vi "Memory Management.MoveDblBlock.Write (Double).vi"(0 "src ptr in":u64, 1 "src offset (0)":u64, 2 "dst in":dbl[](array[numeric]), 3 "dst index (0)":u64, 4 "count":u64, 5 "error in (no error)":errorcluster) -> (14 "src ptr out":u64, 15 "src offset out":u64, 16 "dst out":dbl[](array[numeric]), 17 "dst index out":u64, 18 "count out":u64, 19 "error out":errorcluster)   [LabVIEW 2016, in "VeriStand Data.lvlib"]
uses:
  VeriStand Data.lvlib
  <vilib>/NI Veristand/Custom Device API/data/NIVeriStand_DataServices.dll
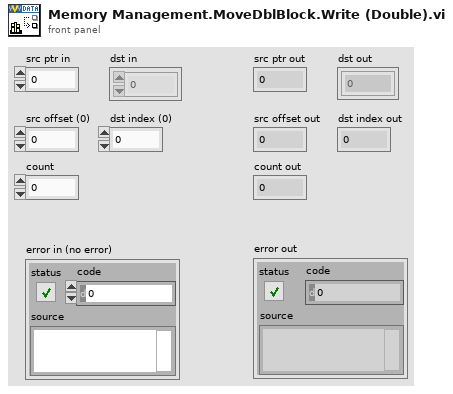
[diagram p1: front panel]
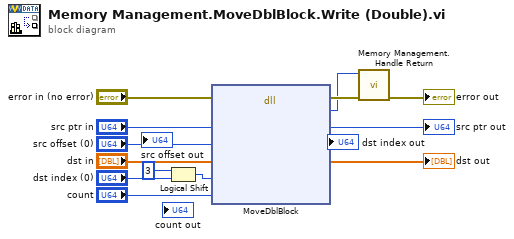
[diagram p0: block diagram]
diagram:
  n1 = Logical Shift(y=i16 3, x="dst index (0)") -> (x << y=w5:u64)
  n2 = dll-call lib="C:/Program Files (x86)/National Instruments/LabVIEW 2016/vi.lib/NI Veristand/Custom Device API/data/NIVeriStand_DataServices.*" fn="MoveDblBlock"(error in="error in (no error)", "srcPtr"="src ptr in", "srcOffset"="src offset (0)", "dstPtr"="dst in", "dstOffset"=w5, "count"="count") -> (error out=w3:errorcluster, "return type"=w1:i32, "srcPtr"=→"src ptr out":u64, "dstPtr"=→"dst out":dbl[])  [unwired: 5 in, 1 out]
  n3 = call "Memory Management.Handle Return.vi"("error in (no error)"=w3, "return"=w1) -> ("error out"=→"error out":errorcluster)  [unwired: 9 in]
